vi "Initialize New Channels.vi"(8 "error in (no error)":errorcluster, 11 "Node Ptr":T4 format="%.0x") -> (0 "error out":errorcluster)   [LabVIEW 2011, in "Simulated Thermocouple Custom Device.lvlib"]
uses:
  Simulated Thermocouple Custom Device.lvlib
  <vilib>/NI Veristand/Custom Device API/Custom Device Item Ref.ctl
  New Channel Data.ctl
  TC Selector.ctl
  TC Unit Selector.ctl
  Device Settings.ctl
  <vilib>/NI Veristand/Custom Device API/Set Item Property (Variant).vi
  <vilib>/NI Veristand/Custom Device API/Custom Device API.lvlib
panel:
  in  "# Channels of the above type":u32
  in  "Channel Count":u32[](array[numeric])=[0, 0, 0, 0, 0, 0, 0, 0] max=32
  in  "Thermocouple Type":T1 items=["J", "K", "T", "E", "N", "B", "R", "S"]
  in  "Temperature Units":T2 items=["Celcius", "Fahrenheit", "Kelvin", "Rankine"]
  in  "Header 2":cluster{"Section Name":string}={"Section Name"="Simulated Thermocouple Channels"}
  in  "Header":cluster{"Section Name":string}={"Section Name"="Auxiliary Channels"}
  in  "Channel Data":T3 {"Device Chan Total" max=32 step=1; "Thermocouple"."Temperature Units" items=["Celcius", "Fahrenheit", "Kelvin", "Rankine", "Volts"]; "Thermocouple"."Thermocouple Type" items=["J", "K", "T", "E", "N", "B", "R", "S", "Raw Voltage"]}
  in  "Device Channel Count":u16(ring)=6 items=["2", "4", "8", "12", "16", "24", "32"]
  in  "Physical Device":string
  in  "Low Side Resistance (Ohms)":dbl=150.0 min=0.1
  in  "High Side Resistance (Ohms)":dbl=15000.0 min=0.1
  in  "# of Current Channels":u32 max=32
  in  "# of Voltage Channels":u32 max=32
  in  "Cancel Button":bool
  in  "OK Button":bool
  # "For each type of thermocouple, select\nthe number of channels to add"
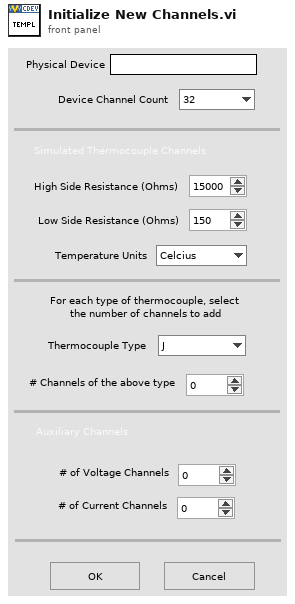
[diagram p1: front panel]
types:
  T1 = typedef "Simulated Thermocouple Custom Device.lvlib/TC Selector.ctl" = u16
  T2 = typedef "Simulated Thermocouple Custom Device.lvlib/TC Unit Selector.ctl" = u16
  T3 = typedef "Simulated Thermocouple Custom Device.lvlib/New Channel Data.ctl" = cluster{"Voltage":u32, "Current":u32, "Thermocouple":cluster{"R1":dbl, "R2":dbl, "Decimation":u32, "Thermocouple Type":T1, "Temperature Units":T2, "Channel Count":u32[]}, "Physical Device":string, "Device Chan Total":u32}
  T4 = typedef "Custom Device API.lvlib/Custom Device Item Ref.ctl" = u64
  T5 = enum8{"Enabled", "Disabled", "Disabled and Grayed Out"}
  T6 = typedef "Simulated Thermocouple Custom Device.lvlib/Device Settings.ctl" = cluster{"High Side Resistance (Ohms)":dbl, "Low Side Resistance (Ohms)":dbl, "Temperature Units":T2, "Update Rate":dbl, "Physical Device Name":string, "Device Channel Count":u32}
  T7 = typedef "Simulated Thermocouple Custom Device.lvlib/Device Config data.ctl" = cluster{"Custom Device Ref":T4, "Voltage Section Ref":T4, "simTC Section Refs":T4[], "Current Section Ref":T4, "Physical Device":string, "Available Physical Channels":i32[], "Channel Counts":u32[], "Dev Chan Count":u32}
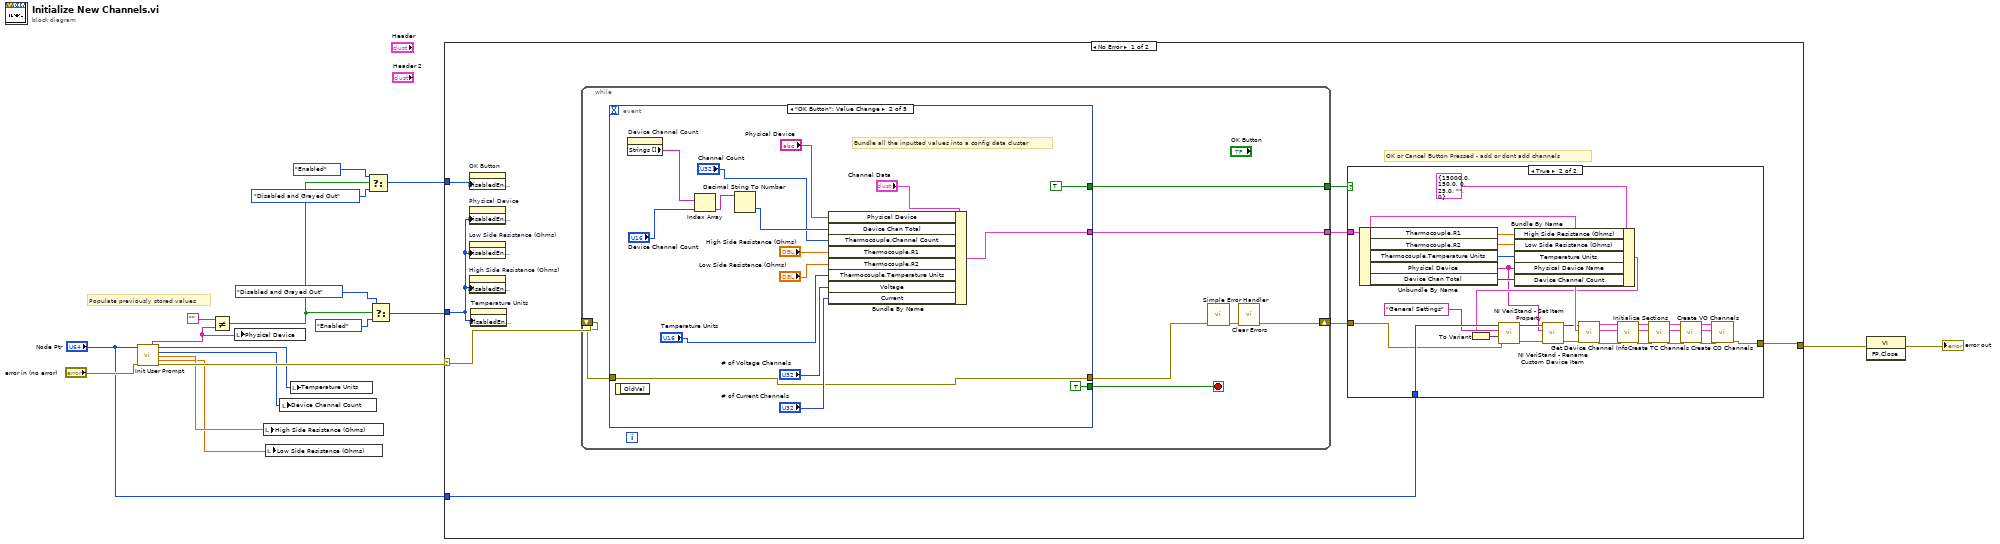
[diagram p0: block diagram]
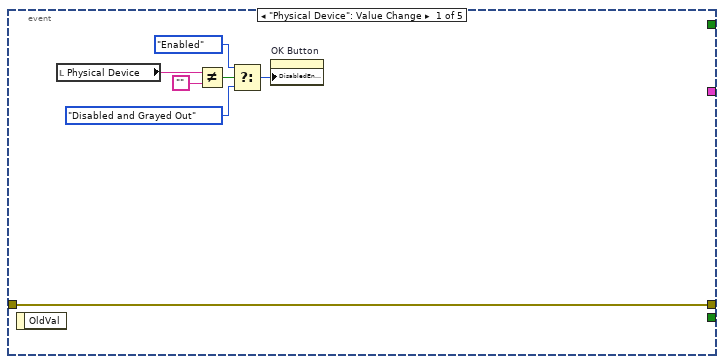
[diagram p3: hidden frame]
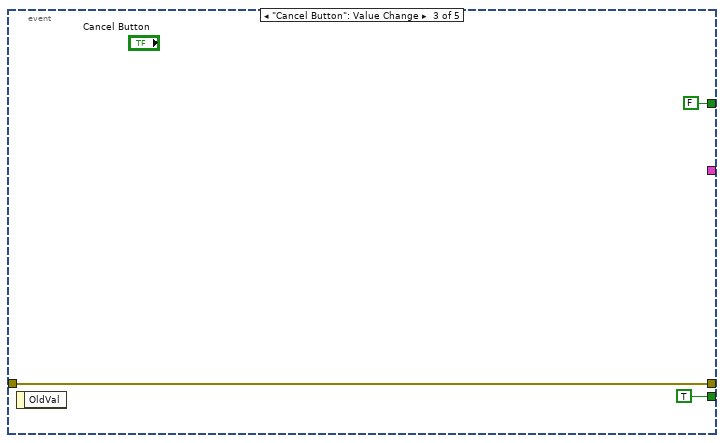
[diagram p4: hidden frame]
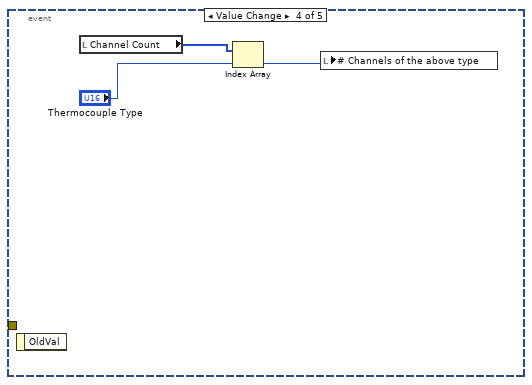
[diagram p5: hidden frame]
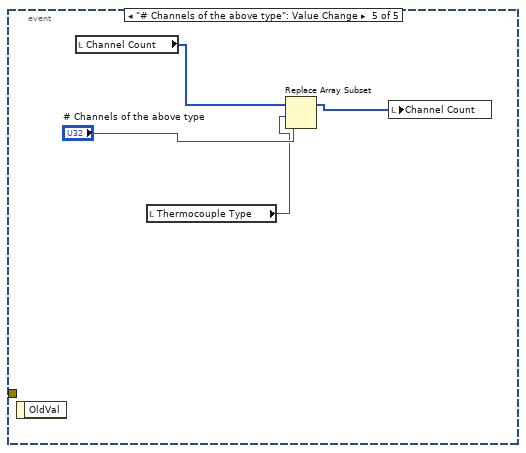
[diagram p6: hidden frame]
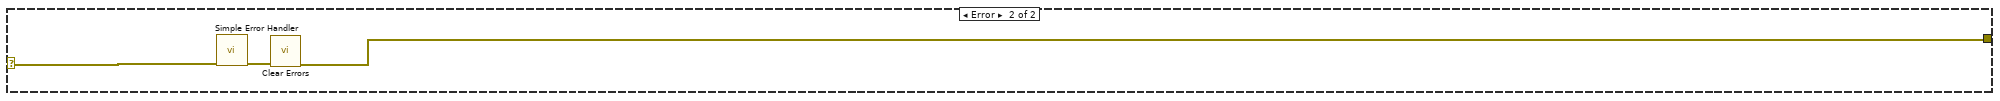
[diagram p7: hidden frame]
diagram:
  # "Populate previously stored values"
  n1 = call "Init User Prompt.vi"("Custom Device Ref in"="Node Ptr", "error in"="error in (no error)") -> ("Physical Device Name"=w2:string, "Temperature Units"=w1:T2, "Dev Chan Count"=w6:u32, "High Side Resistor"=w5:dbl, "Low Side Resistor"=w4:dbl, "error out"=w9:errorcluster)  [unwired: 8 in]
  n2 = Not Equal?(x="", y=w2) -> (x != y?=w3:bool)
  n3 = local write "Physical Device"(w2) -> ()
  n4 = local write "High Side Resistance (Ohms)"(w5) -> ()
  n5 = local write "Low Side Resistance (Ohms)"(w4) -> ()
  n6 = local write "Device Channel Count"(w6) -> ()
  n7 = local write "Temperature Units"(w1) -> ()
  n8 = Select(t=T5."Enabled" ("Disabled"), s=w3, f=T5."Disabled and Grayed Out" ("Disabled")) -> (s? t:f=w12:T5)
  n9 = Select(t=T5."Disabled and Grayed Out" ("Disabled"), s=w3, f=T5."Enabled" ("Disabled")) -> (s? t:f=w15:T5)
  n10 = case shown="No Error" w9 {
    selector: w9 -> [w26 w99]
    tunnel: [w24 w97] -> w18
    tunnel: w15 -> [w19 _]
    tunnel: "Node Ptr" -> [w21 _]
    tunnel: w12 -> [w25 _]
    frame No Error {
      # "OK or Cancel Button Pressed - add or dont add channels"
      n11 = property on="OK Button" class="Bool"("DisabledEnum"=w25) -> ()  [unwired: 2 in, 2 out]
      n12 = property on="Physical Device" class="Str"("DisabledEnum"=w19) -> ()  [unwired: 2 in, 2 out]
      n13 = property on="Low Side Resistance (Ohms)" class="DigNum (strict)"("DisabledEnum"=w19) -> ()  [unwired: 2 in, 2 out]
      n14 = property on="High Side Resistance (Ohms)" class="DigNum (strict)"("DisabledEnum"=w19) -> ()  [unwired: 2 in, 2 out]
      n15 = property on="Temperature Units" class="Ring (strict)"("DisabledEnum"=w19) -> ()  [unwired: 2 in, 2 out]
      n16 = while {
        shift-right: [w59] -> w23
        shift-left: w26 -> [w63]
        tunnel: [w58] -> w22
        tunnel: [w57] -> w20
        stop <- w62 stop-if-true
        n17 = event shown="[1] \"OK Button\": Value Change" {
          selector: _ -> [_ _ _ _ _]
          dyn-events: _ -> [_ _ _ _ _]
          timeout: _ -> [_ _ _ _ _]
          tunnel: w63 -> [w64 w74 w88 _ _]
          tunnel: [_ TRUE TRUE _ _] -> w62
          tunnel: [w64 w74 w88 _ _] -> w61
          tunnel: [_ w81 _ _ _] -> w58
          tunnel: [_ TRUE FALSE _ _] -> w57
          event "Physical Device": Value Change {
            n18 = event-data() -> ()  [unwired: 2 out]
            n19 = local read "Physical Device"() -> (w66:string)
            n20 = Not Equal?(x=w66, y="") -> (x != y?=w67:bool)
            n21 = Select(t=T5."Enabled" ("Disabled"), s=w67, f=T5."Disabled and Grayed Out" ("Disabled")) -> (s? t:f=w70:T5)
            n22 = property on="OK Button" class="Bool"("DisabledEnum"=w70) -> ()  [unwired: 2 in, 2 out]
          }
          event "OK Button": Value Change {
            # "Bundle all the inputted values into a config data cluster"
            n23 = event-data() -> ()  [unwired: 2 out]
            n24 = property on="Device Channel Count" class="Ring (strict)"() -> ("Strings []"=w78:string[])  [unwired: 2 in, 2 out]
            n25 = Index Array(array=w78, index="Device Channel Count") -> (element=w76:string)
            n26 = Decimal String To Number(string=w76) -> (number=w75:i32)  [unwired: 2 in, 1 out]
            n27 = Bundle By Name(cluster="Channel Data", "Physical Device"="Physical Device", "Device Chan Total"=w75, "Thermocouple.Channel Count"="Channel Count", "Thermocouple.R1"="High Side Resistance (Ohms)", "Thermocouple.R2"="Low Side Resistance (Ohms)", "Thermocouple.Temperature Units"="Temperature Units", "Voltage"="# of Voltage Channels", "Current"="# of Current Channels") -> (w81:T3)
          }
          event "Cancel Button": Value Change {
            n28 = event-data() -> ()  [unwired: 2 out]
          }
          event Value Change {
            n29 = event-data() -> ()  [unwired: 2 out]
            n30 = local read "Channel Count"() -> (w92:u32[])
            n31 = Index Array(array=w92, index="Thermocouple Type") -> (element=w90:u32)
            n32 = local write "# Channels of the above type"(w90) -> ()
          }
          event "# Channels of the above type": Value Change {
            n33 = event-data() -> ()  [unwired: 2 out]
            n34 = local read "Channel Count"() -> (w96:u32[])
            n35 = local read "Thermocouple Type"() -> (w94:T1)
            n36 = Replace Array Subset(array=w96, new element="# Channels of the above type", index=w94) -> (w93:u32[])
            n37 = local write "Channel Count"(w93) -> ()
          }
        }
        n38 = call <vilib>:"Simple Error Handler.vi"("error in (no error)"=w61) -> ("error out"=w60:errorcluster)  [unwired: 1 in, 7 out]
        n39 = call <vilib>:"Clear Errors.vi"("error in (no error)"=w60) -> ("error out"=w59:errorcluster)  [unwired: 6 out]
      }
      n40 = case shown="True" w20 {
        tunnel: [w27 w31] -> w24
        tunnel: w23 -> [w27 w34]
        tunnel: w22 -> [_ w44]
        tunnel: w21 -> [_ w43]
        frame False {
        }
        frame True {
          n41 = Unbundle By Name(w44) -> ("Thermocouple.R1"=w41:dbl, "Thermocouple.R2"=w40:dbl, "Thermocouple.Temperature Units"=w39:T2, "Physical Device"=w32:string, "Device Chan Total"=w38:u32)
          n42 = Bundle By Name(cluster=T6 {"High Side Resistance (Ohms)"=15000.0, "Low Side Resistance (Ohms)"=150.0, "Temperature Units"=0, "Update Rate"=25.0, "Physical Device Name"="", "Device Channel Count"=0} ("General Settings"), "High Side Resistance (Ohms)"=w41, "Low Side Resistance (Ohms)"=w40, "Temperature Units"=w39, "Physical Device Name"=w32, "Device Channel Count"=w38) -> (w35:T6)
          n43 = To Variant(anything=w35) -> (Variant=w36:variant)
          n44 = call-poly <vilib>:"NI VeriStand - Set Item Property.vi"("error in (no error)"=w34, "Value"=w36, "Property Name"="General Settings", "Item Ref in"=w43) -> ("error out"=w29:errorcluster, "Item Ref out"=w33:T4)  [unwired: 5 in, 1 out]
          n45 = call <vilib>:"NI VeriStand - Rename Custom Device Item.vi"("error in (no error)"=w29, "New Name"=w32, "Item Ref in"=w33) -> ("error out"=w30:errorcluster, "Item Ref out"=w28:T4)  [unwired: 6 in, 1 out]
          n46 = call "Get Device Channel Info.vi"("error in"=w30, "Channel Data in"=w44, "Custom Device Ref in"=w28) -> ("error out"=w56:errorcluster, "Channel Data out"=w54:T3, "Device Configuration Data"=w55:T7)  [unwired: 6 in]
          n47 = call "Initialize Sections.vi"("Device Configuration Data In"=w55, "Channel Data In"=w54, "error in (no error)"=w56) -> ("Device Configuration Data  Out"=w53:T7, "Channel Data Out"=w50:T3, "error Out (no error)"=w47:errorcluster)  [unwired: 5 in]
          n48 = call "Create TC Channels.vi"("error in"=w47, "Channel Data in"=w50, "Device Configuration Data In"=w53) -> ("error out"=w46:errorcluster, "Channel Data Out"=w49:T3, "Device Configuration Data Out"=w52:T7)  [unwired: 6 in]
          n49 = call "Create VO Channels.vi"("error in"=w46, "Channel Data in"=w49, "Device Configuration Data In"=w52) -> ("error out"=w45:errorcluster, "Channel Data Out"=w48:T3, "Device Configuration Data Out"=w51:T7)  [unwired: 6 in]
          n50 = call "Create CO Channels.vi"("error in"=w45, "Channel Data in"=w48, "Device Configuration Data In"=w51) -> ("error out"=w31:errorcluster)  [unwired: 6 in, 2 out]
        }
      }
    }
    frame Error {
      n51 = call <vilib>:"Simple Error Handler.vi"("error in (no error)"=w99) -> ("error out"=w98:errorcluster)  [unwired: 1 in, 7 out]
      n52 = call <vilib>:"Clear Errors.vi"("error in (no error)"=w98) -> ("error out"=w97:errorcluster)  [unwired: 6 out]
    }
  }
  n53 = invoke class="VI" method="FP.Close"(error in=w18) -> (error out=→"error out":errorcluster)  [unwired: 2 in, 2 out]
